vi "Calculate Channel Value.vi"(9 "Digital":bool=TRUE, 10 "Remaining Time":dbl, 11 "Step Settings":T1) -> (3 "Values to Write":dbl[](array[numeric]))   [LabVIEW 2020, in "Sequencer with Output Values.lvlib" / "Sequencer with Output Values.lvclass"]
uses:
  Sequencer with Output Values.lvclass
  Step Settings.ctl
  Global Strings.vi
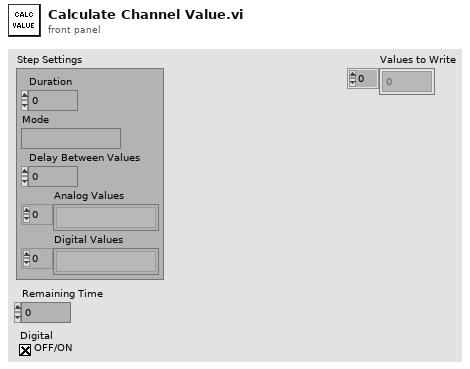
[diagram p1: front panel]
types:
  T1 = typedef "Step Settings.ctl" = cluster{"Duration":dbl, "Mode":string, "Delay Between Values":dbl, "Analog Values":string[], "Digital Values":string[]}
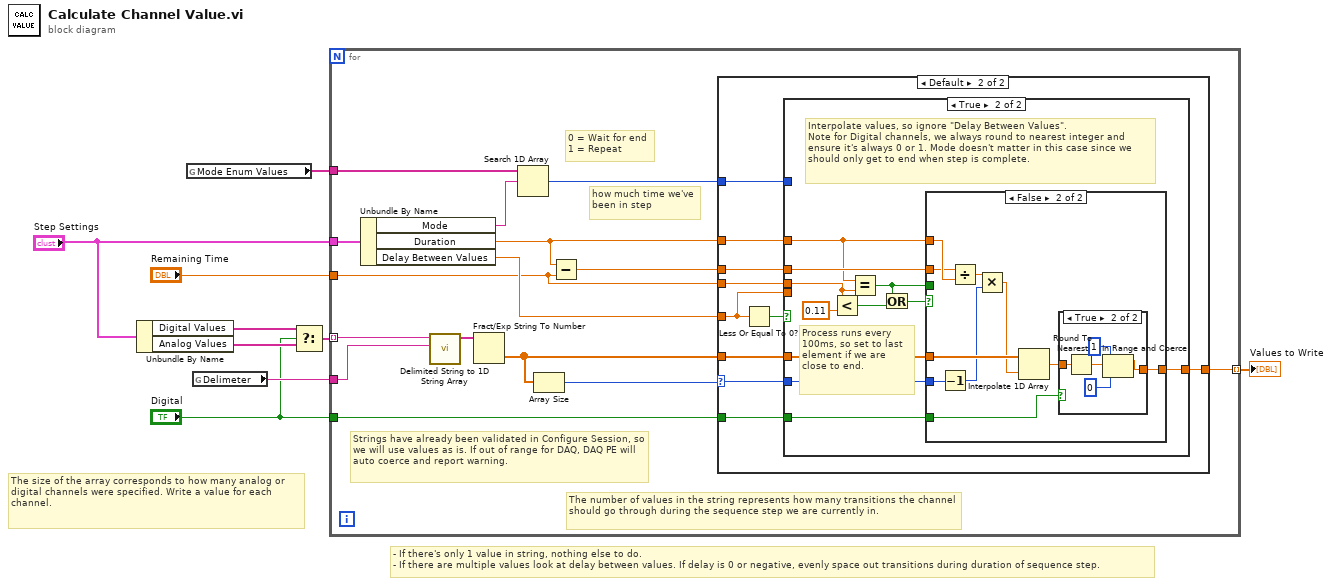
[diagram p0: block diagram]
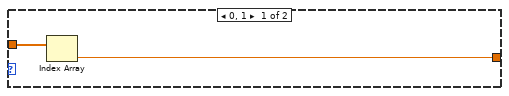
[diagram p2: hidden frame]
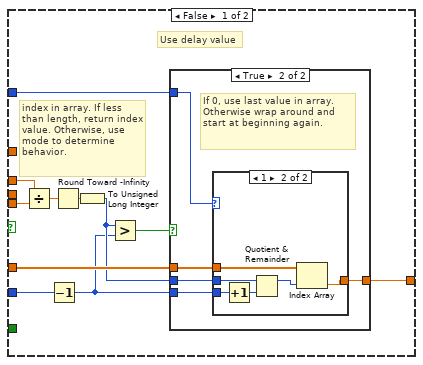
[diagram p3: hidden frame]
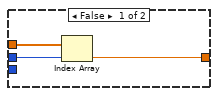
[diagram p4: hidden frame]
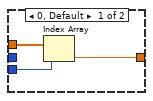
[diagram p5: hidden frame]
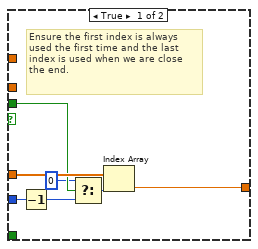
[diagram p6: hidden frame]
diagram:
  # "The size of the array corresponds to how many analog or digital channels were specified. Write a value for each channel."
  # "- If there's only 1 value in string, nothing else to do. \n- If there are multiple values look at delay between values. If delay is 0 or negative, evenly space out transitions during duration of sequence step."
  n1 = Unbundle By Name("Step Settings") -> ("Digital Values"=w5:string[], "Analog Values"=w4:string[])
  n2 = global read "Global Strings.vi" "Mode Enum Values"() -> (w7:string[])
  n3 = global read "Global Strings.vi" "Delimeter"() -> (w9:string)
  n4 = Select(t=w5, s="Digital", f=w4) -> (s? t:f=w1:string[])
  n5 = for {
    tunnel: w1 -> [w24] mode=indexing
    tunnel: w9 -> [w23]
    tunnel: "Digital" -> [w18]
    tunnel: "Step Settings" -> [w17]
    tunnel: "Remaining Time" -> [w14]
    tunnel: w7 -> [w13]
    tunnel: [w10] -> w2 mode=indexing
    # "The number of values in the string represents how many transitions the channel should go through during the sequence step we are currently in."
    # "Strings have already been validated in Configure Session, so we will use values as is. If out of range for DAQ, DAQ PE will auto coerce and report warning."
    # "how much time we've been in step"
    # "0 = Wait for end\n1 = Repeat"
    n6 = Unbundle By Name(w17) -> ("Mode"=w12:string, "Duration"=w16:dbl, "Delay Between Values"=w15:dbl)
    n7 = call <vilib>:"Delimited String to 1D String Array.vi"("delimiter"=w23, "delimited string"=w24) -> ("string array"=w22:string[])  [unwired: 9 in]
    n8 = Fract/Exp String To Number(string=w22) -> (number=w19:dbl[])  [unwired: 3 in, 1 out]
    n9 = Search 1D Array(1D array=w13, element=w12) -> (index of element=w11:i32)  [unwired: 1 in]
    n10 = Array Size(array=w19) -> (size(s)=w20:i32)
    n11 = Subtract(x=w16, y=w14) -> (x-y=w21:dbl)
    n12 = case shown="Default" w20 {
      selector: w20 -> [_ w31]
      tunnel: w19 -> [w26 w35]
      tunnel: [w25 w30] -> w10
      tunnel: w15 -> [_ w33]
      tunnel: w21 -> [_ w34]
      tunnel: w11 -> [_ w32]
      tunnel: w16 -> [_ w29]
      tunnel: w18 -> [_ w28]
      tunnel: w14 -> [_ w27]
      frame 0, 1 {
        n13 = Index Array(array=w26) -> (element=w25:dbl)  [unwired: 1 in]
      }
      frame Default {
        n14 = Less Or Equal To 0?(x=w33) -> (x <= 0?=w36:bool)
        n15 = case shown="True" w36 {
          tunnel: w35 -> [w42 w75]
          tunnel: w34 -> [w47 w73]
          tunnel: w33 -> [w46 _]
          tunnel: w32 -> [w38 _]
          tunnel: w31 -> [w44 w74]
          tunnel: [w39 w72] -> w30
          tunnel: w29 -> [_ w68]
          tunnel: w28 -> [_ w65]
          tunnel: w27 -> [_ w69]
          frame False {
            # "Use delay value"
            # "index in array. If less than length, return index value. Otherwise, use mode to determine behavior."
            n16 = Divide(x=w47, y=w46) -> (x/y=w45:dbl)
            n17 = Decrement(x=w44) -> (x-1=w37:i32)
            n18 = Round Toward -Infinity(1:w45) -> (0:w41:dbl)
            n19 = To Unsigned Long Integer(number=w41) -> (unsigned 32bit integer=w40:u32)
            n20 = Greater?(x=w40, y=w37) -> (0:w43:bool)
            n21 = case shown="True" w43 {
              tunnel: w42 -> [w50 w54]
              tunnel: w40 -> [w49 w51]
              tunnel: [w48 w52] -> w39
              tunnel: w38 -> [_ w55]
              tunnel: w37 -> [_ w53]
              frame False {
                n22 = Index Array(array=w50, index=w49) -> (element=w48:dbl)
              }
              frame True {
                # "If 0, use last value in array. Otherwise wrap around and start at beginning again."
                n23 = case shown="1" w55 {
                  tunnel: w54 -> [w58 w63]
                  tunnel: w53 -> [w57 w60]
                  tunnel: [w56 w61] -> w52
                  tunnel: w51 -> [_ w64]
                  frame 0, Default {
                    n24 = Index Array(array=w58, index=w57) -> (element=w56:dbl)
                  }
                  frame 1 {
                    n25 = Increment(x=w60) -> (x+1=w59:i32)
                    n26 = Quotient & Remainder(x=w64, y=w59) -> (x-y*floor(x/y)=w62:u32)  [unwired: 1 out]
                    n27 = Index Array(array=w63, index=w62) -> (element=w61:dbl)
                  }
                }
              }
            }
          }
          frame True {
            # "Process runs every 100ms, so set to last element if we are close to end."
            # "Interpolate values, so ignore \"Delay Between Values\". \nNote for Digital channels, we always round to nearest integer and ensure it's always 0 or 1. Mode doesn't matter in this case since we should only get to end when step is complete."
            n28 = Less?(x=w69, y=0.11) -> (x < y?=w70:bool)
            n29 = Equal?(x=w68, y=w69) -> (x = y?=w66:bool)
            n30 = Or(x=w66, y=w70) -> (x .or. y?=w67:bool)
            n31 = case shown="False" w67 {
              tunnel: w75 -> [w82 w92]
              tunnel: w74 -> [w81 w90]
              tunnel: w68 -> [_ w87]
              tunnel: w73 -> [_ w86]
              tunnel: [w78 w83] -> w72
              tunnel: w66 -> [w80 _]
              tunnel: w65 -> [_ w85]
              frame True {
                # "Ensure the first index is always used the first time and the last index is used when we are close the end."
                n32 = Decrement(x=w81) -> (x-1=w76:i32)
                n33 = Select(t=0 ("f"), s=w80, f=w76) -> (s? t:f=w79:i32)
                n34 = Index Array(array=w82, index=w79) -> (element=w78:dbl)
              }
              frame False {
                n35 = Decrement(x=w90) -> (x-1=w89:i32)
                n36 = Divide(x=w86, y=w87) -> (x/y=w91:dbl)
                n37 = Multiply(x=w91, y=w89) -> (x*y=w88:dbl)
                n38 = Interpolate 1D Array(1:w88, 2:w92) -> (0:w84:dbl)
                n39 = case shown="True" w85 {
                  tunnel: w84 -> [w93 w98]
                  tunnel: [w93 w96] -> w83
                  frame False {
                  }
                  frame True {
                    n40 = Round To Nearest(number=w98) -> (nearest integer value=w97:dbl)
                    n41 = In Range and Coerce(upper limit=1, x=w97, lower limit=0) -> (coerced(x)=w96:dbl)  [unwired: 1 out]
                  }
                }
              }
            }
          }
        }
      }
    }
  }
  "Values to Write" <- w2
